vi "Create.vi"(7 "gRPC server id":T1, 8 "error in (no error)":errorcluster, 9 "IMeasurementService in":refnum<class "IMeasurement Service.lvclass">, 10 "MeasurementPluginService in":refnum<class "Measurement Plugin Service.lvclass">, 11 "pin map context":T2) -> (0 "error out":errorcluster, 3 "MeasurementContext out":refnum<class "Measure Call Context.lvclass">)   [LabVIEW 2020, in "MeasurementLink Measurement Server.lvlib" / "Measure Call Context.lvclass"]
uses:
  Measure Call Context.lvclass
  Helpers/TypeDefs/PinMapContext.ctl
  <vilib>/gRPC/LabVIEW gRPC Library/Shared/grpcId.ctl
  IMeasurement Service/IMeasurement Service.lvclass
  Measurement Plugin Service/Measurement Plugin Service.lvclass
  Data.ctl
  MeasurementLink Session Management Client/RPC Messages/ni_measurementlink_sessionmanagement_v1_SessionInformation.ctl
  MeasurementLink Session Management Client/RPC Messages/nidevice_grpc_Session.ctl
  MeasurementLink Session Management Client/RPC Messages/ni_measurementlink_sessionmanagement_v1_ChannelMapping.ctl
  Measure Call Context.lvclass/Measure Call Context.ctl
  MeasurementLink Measurement Server.lvlib
  <vilib>/gRPC/LabVIEW gRPC Library/grpc-lvsupport-release.lvlib
  MeasurementLink Session Management Client/MeasurementLink Session Management Client.lvlib
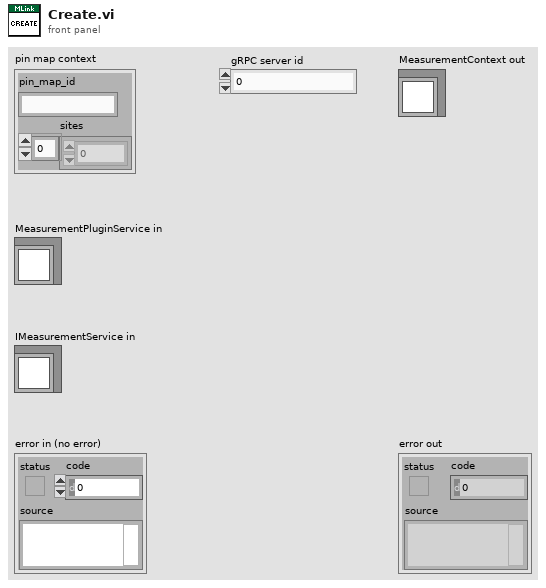
[diagram p1: front panel]
types:
  T1 = typedef "grpc-lvsupport-release.lvlib/grpcId.ctl" = u64
  T2 = typedef "MeasurementLink Measurement Server.lvlib/PinMapContext.ctl" = cluster{"pin_map_id":string, "sites":i32[]}
  T3 = typedef "MeasurementLink Measurement Server.lvlib/Measure Call Context.lvclass/Data.ctl" = cluster{"PinMapContext":T2, "gRPCServerId":T1, "IMeasurementService":refnum<class "IMeasurement Service.lvclass">, "MeasurementPluginService":refnum<class "Measurement Plugin Service.lvclass">, "reserved session infos":set{T4}}
  T4 = typedef "MeasurementLink Session Management Client.lvlib/ni_measurementlink_sessionmanagement_v1_SessionInformation.ctl" = cluster{"session":T5, "resource_name":string, "channel_list":string, "instrument_type_id":string, "session_exists":bool, "channel_mappings":T6[]}
  T5 = typedef "MeasurementLink Session Management Client.lvlib/nidevice_grpc_Session.ctl" = cluster{"name":string}
  T6 = typedef "MeasurementLink Session Management Client.lvlib/ni_measurementlink_sessionmanagement_v1_ChannelMapping.ctl" = cluster{"pin_or_relay_name":string, "site":i32, "channel":string}
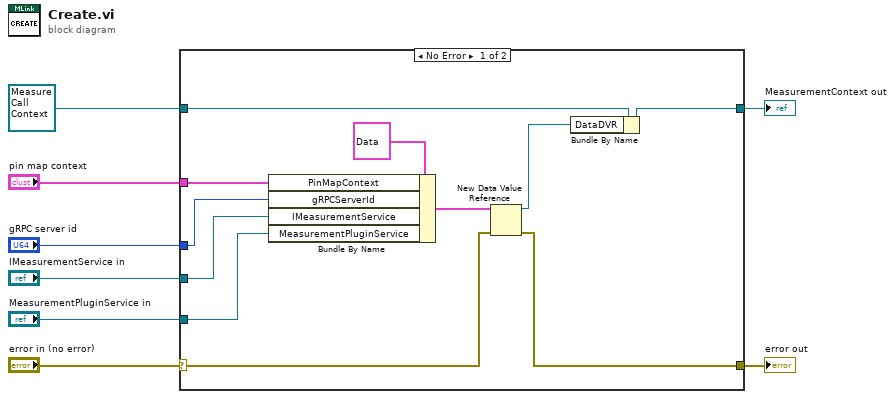
[diagram p0: block diagram]
diagram:
  n1 = case shown="No Error" "error in (no error)" {
    selector: "error in (no error)" -> [w12 w21]
    tunnel: [w9 w21] -> w7
    tunnel: [w18 w20] -> w6
    tunnel: refnum<class "Measure Call Context.lvclass"> refnum ("MeasurementContext.lvclass") -> [w19 w20]
    tunnel: "pin map context" -> [w16 _]
    tunnel: "gRPC server id" -> [w15 _]
    tunnel: "IMeasurementService in" -> [w14 _]
    tunnel: "MeasurementPluginService in" -> [w13 _]
    frame No Error {
      n2 = Bundle By Name(cluster=T3 {"PinMapContext"={"pin_map_id"="", "sites"=[]}, "gRPCServerId"=0, "IMeasurementService"=refnum, "MeasurementPluginService"=refnum, "reserved session infos"={}} ("Data"), "PinMapContext"=w16, "gRPCServerId"=w15, "IMeasurementService"=w14, "MeasurementPluginService"=w13) -> (w11:T3)
      n3 = New Data Value Reference(data value=w11, error in=w12) -> (data value reference=w10:refnum<data-value>, error out=w9:errorcluster)
      n4 = Bundle By Name(cluster=w19, "DataDVR"=w10) -> (w18:refnum<class "Measure Call Context.lvclass">)
    }
    frame Error {
    }
  }
  "error out" <- w7
  "MeasurementContext out" <- w6
